vi "Autonomous Independent.vi"() -> ()   [LabVIEW 2016]
doc: "This VI is called when autonomous begins, and will automatically be terminated when autonomous ends. You can carry out timed or sensor driven robot movement independently without needing to return to the caller."
uses:
  <vilib>/Rock Robotics/WPI/Solenoid/WPI_SolenoidValue.ctl
  <vilib>/Rock Robotics/WPI/SafetyOutput/WPI_SafetyOutputConfigMenu.ctl
  <vilib>/Rock Robotics/WPI/Utilities/WPI_GetSetVariantRefNum.vi
  <vilib>/Rock Robotics/Network Tables/NT Read String.vi
  <vilib>/Rock Robotics/Network Tables/NT Write Numeric Array.vi
  <vilib>/Rock Robotics/WPI/Ultrasonic/WPI_SonarMB1010AnalogRefNum Registry Get.vi
  <vilib>/Rock Robotics/WPI/RobotDrive/WPI_RobotDriveArcadeDrive_Standard(NoSaturation).vi
  <vilib>/Rock Robotics/WPI/Solenoid/WPI_SolenoidSetEnum.vi
  <vilib>/addons/control/pid/pid.llb/PID (DBL).vi
  <vilib>/Rock Robotics/WPI/Ultrasonic/WPI_SonarMB1010AnalogGetRange.vi
  <vilib>/Rock Robotics/WPI/ThirdParty/Sensors/ADIS16448 IMU/ADIS16448_IMU.lvlib
  <vilib>/addons/control/pid/NI_PID_pid.lvlib
panel:
  out "Current Movement, for debugging":T1 {"Y Joystick Value" scale=1.0..-1.0; "X Joystick Value" scale=-1.0..1.0}
  in  "Array of robot movements":T2(array[cluster])=[{"X Joystick Value"=0.39393939393939403, "Y Joystick Value"=0.0, "Delay (sec)"=1.0, "Movement Name"="turn"}, {"X Joystick Value"=-0.3737373737373737, "Y Joystick Value"=0.0, "Delay (sec)"=1.0, "Movement Name"="turn back"}] {"Y Joystick Value" scale=1.0..-1.0; "X Joystick Value" scale=-1.0..1.0}
  # "Be sure to right-click and choose Data Operations>>Make Current Value default if you want to save the array values with the VI"
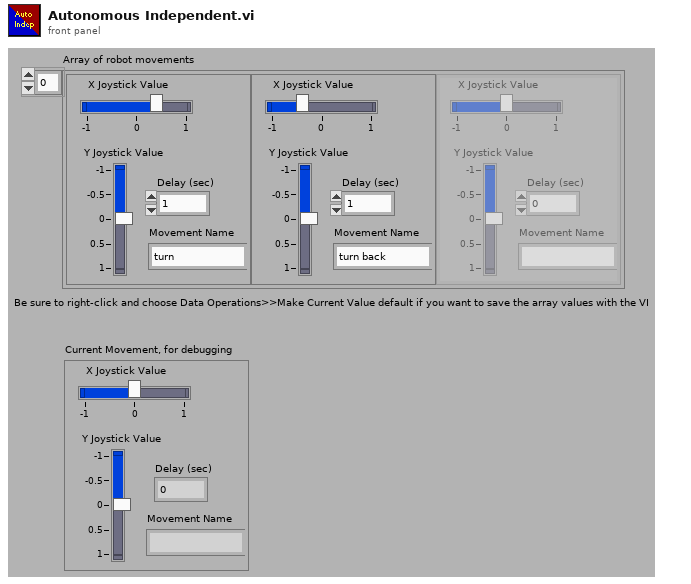
[diagram p1: front panel]
types:
  T1 = cluster{"X Joystick Value":dbl, "Y Joystick Value":dbl, "Delay (sec)":dbl, "Movement Name":string}
  T2 = cluster{"X Joystick Value":dbl, "Y Joystick Value":dbl, "Delay (sec)":dbl, "Movement Name":string}[]
  T3 = typedef "WPI_JoystickDevRef.ctl" = cluster{"Device":T4}
  T4 = typedef "WPI_JoystickDeviceEnum.ctl" = enum16{"USB 0", "USB 1", "USB 2", "USB 3", "USB 4", "USB 5"}
  T5 = typedef "WPI_RobotDriveDevRef.ctl" = cluster{"DevStatus":errorcluster, "Motors[]":T6[], "Square Inputs":bool, "Max Output":dbl}
  T6 = typedef "WPI_MotorControlDeviceRef.ctl" = cluster{"DeviceStatus":errorcluster, "Type":T7, "PWM":cluster{"PWM Channel":T8, "DeadBand":T9}, "CAN":cluster{"Device Number":u8, "SetOutput VI Ref":variant, "GetOutput VI Ref":variant, "Enable VI Ref":variant, "Disable VI Ref":variant, "Data":variant}, "Invert":bool}
  T7 = typedef "WPI_MotorControlType.ctl" = enum16{"PWM", "CAN"}
  T8 = typedef "FPGA_DIOPWMChannel.ctl" = enum8{"PWM 0", "PWM 1", "PWM 2", "PWM 3", "PWM 4", "PWM 5", "PWM 6", "PWM 7", "PWM 8", "PWM 9", "PWM MXP 0", "PWM MXP 1", "PWM MXP 2", "PWM MXP 3", "PWM MXP 4", "PWM MXP 5", "PWM MXP 6", "PWM MXP 7", "PWM MXP 8", "PWM MXP 9", "Invalid"}
  T9 = typedef "WPI_PWMDeadband.ctl" = cluster{"Name":string, "maxPositivePwm":i32, "minPositivePwm":i32, "centerPwm":i32, "maxNegativePwm":i32, "minNegativePwm":i32, "angularRange":u16}
  T10 = typedef "WPI_SonarMB1010AnalogDeviceRef.ctl" = cluster{"AIDeviceRef":T11, "Scaling factor (V/in)":dbl, "Average Bits":u8}
  T11 = typedef "WPI_AnalogChannelDevRef.ctl" = cluster{"DevStatus":errorcluster, "Analog Channel":T12}
  T12 = typedef "FPGA_AIChannel.ctl" = enum8{"AI 0", "AI 1", "AI 2", "AI 3", "AI MXP 0", "AI MXP 1", "AI MXP 2", "AI MXP 3", "Invalid"}
  T13 = typedef "WPI_SolenoidDevRef.ctl" = cluster{"DevStatus":errorcluster, "Pneumatics Control Module":u8, "Forward Solenoid Channel":T14, "Reverse Solenoid Channel":T14}
  T14 = typedef "WPI_SolenoidChannel.ctl" = enum8{"Solenoid 0", "Solenoid 1", "Solenoid 2", "Solenoid 3", "Solenoid 4", "Solenoid 5", "Solenoid 6", "Solenoid 7", "Invalid"}
  T15 = typedef "ADIS16448_IMU.lvlib/ADI_IMU_ADIS16448_InterruptDevRef.ctl" = cluster{"ADI IMU DevRef":T16, "InterruptRef":T18}
  T16 = typedef "ADIS16448_IMU.lvlib/ADI_IMU_ADIS16448_IMUDevRef.ctl" = cluster{"DevStatus":errorcluster, "Handle":i32, "SPI Bus":T17, "Device Found":bool, "Device Ready":bool, "Yaw Axis":enum16{"X", "Y", "Z"}, "AHRS Algorithm":enum16{"Complementary", "Madgwick"}, "Serial":u16, "Lot ID 2":u16, "Lot ID 1":u16, "Product ID":u16}
  T17 = typedef "spi_bus.ctl" = enum16{"SPI On-Board, CS0", "SPI On-Board, CS1", "SPI On-Board, CS2", "SPI On-Board, CS3", "SPI MXP", "Invalid"}
  T18 = typedef "WPI_InterruptRef.ctl" = cluster{"DevStatus":errorcluster, "InterruptIndex":T19}
  T19 = typedef "FPGA_InterruptIndex.ctl" = enum8{"0", "1", "2", "3", "4", "5", "6", "7", "Invalid"}
  T20 = typedef "WPI_SolenoidValue.ctl" = enum16{"Off", "On", "Forward", "Reverse"}
  T21 = typedef "WPI_SafetyOutputConfigMenu.ctl" = enum16{"Enable", "Disable"}
  T22 = cluster{"proportional gain (Kc)":dbl, "integral time (Ti, min)":dbl, "derivative time (Td, min)":dbl}
  T23 = cluster{"X Angle":dbl, "Y Angle":dbl, "Z Angle":dbl}
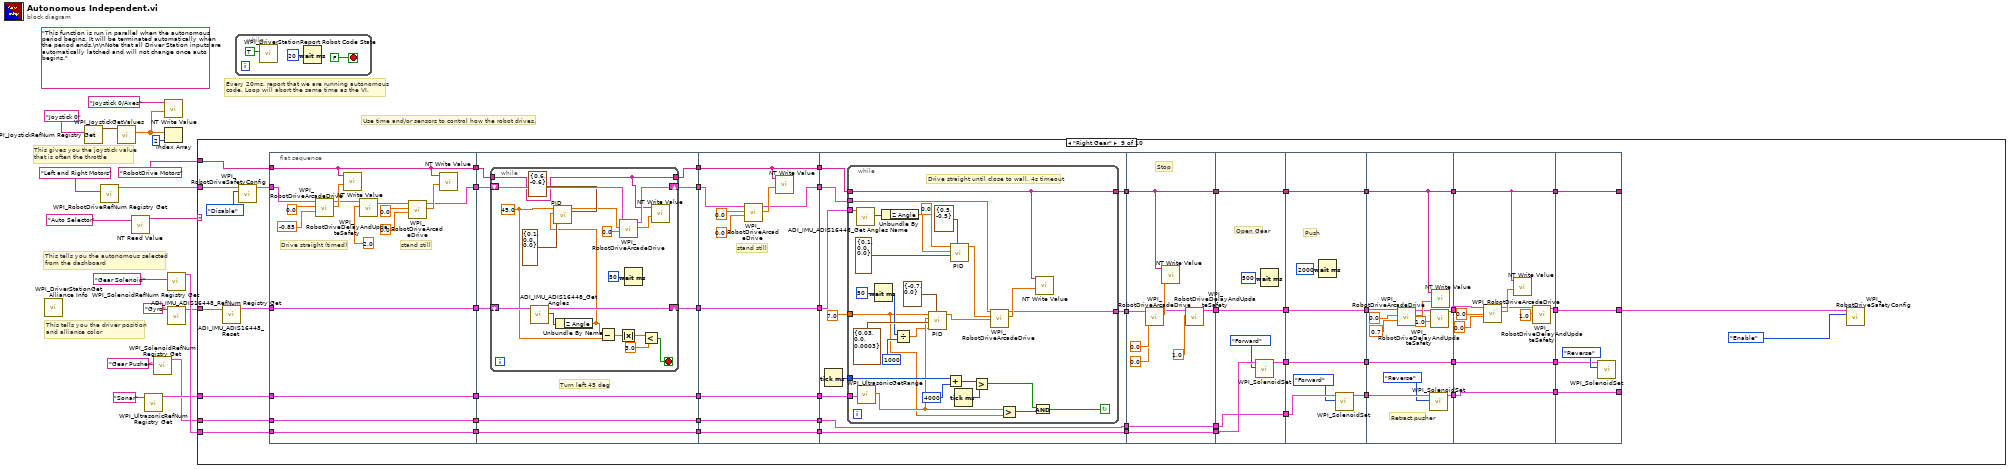
[diagram p0: block diagram]
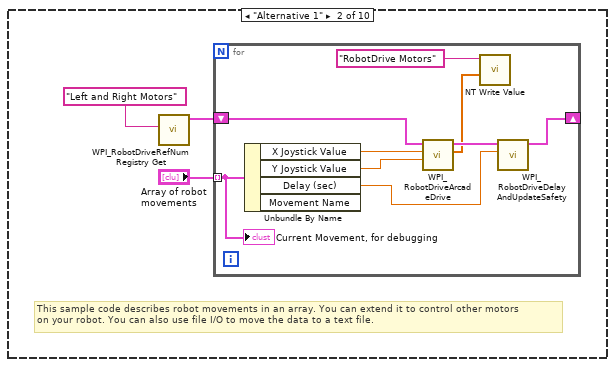
[diagram p3: hidden frame]
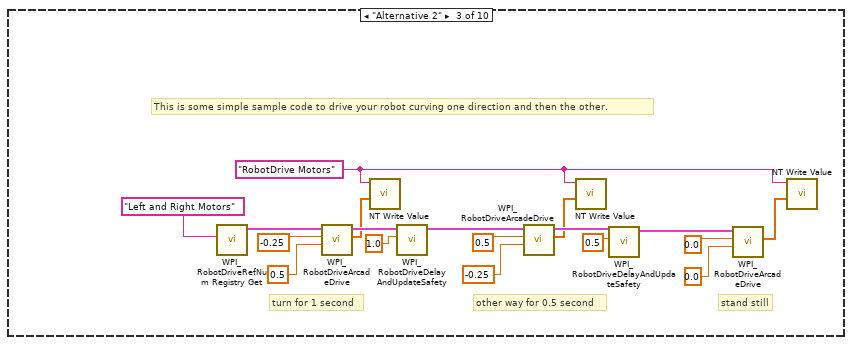
[diagram p4: hidden frame]
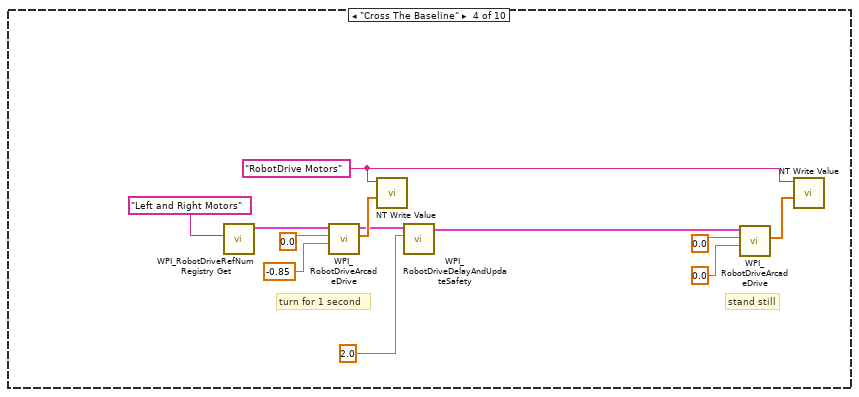
[diagram p5: hidden frame]
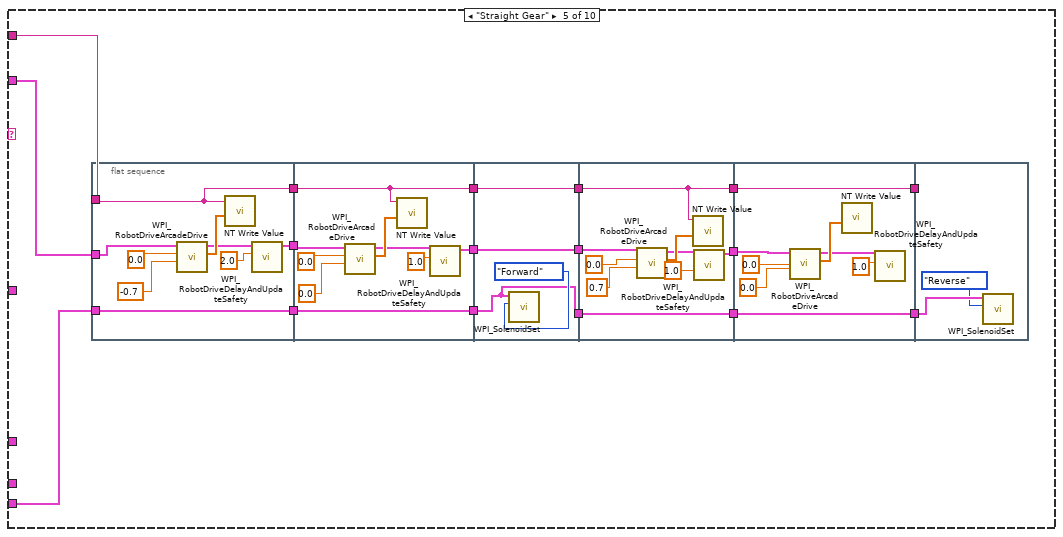
[diagram p6: hidden frame]
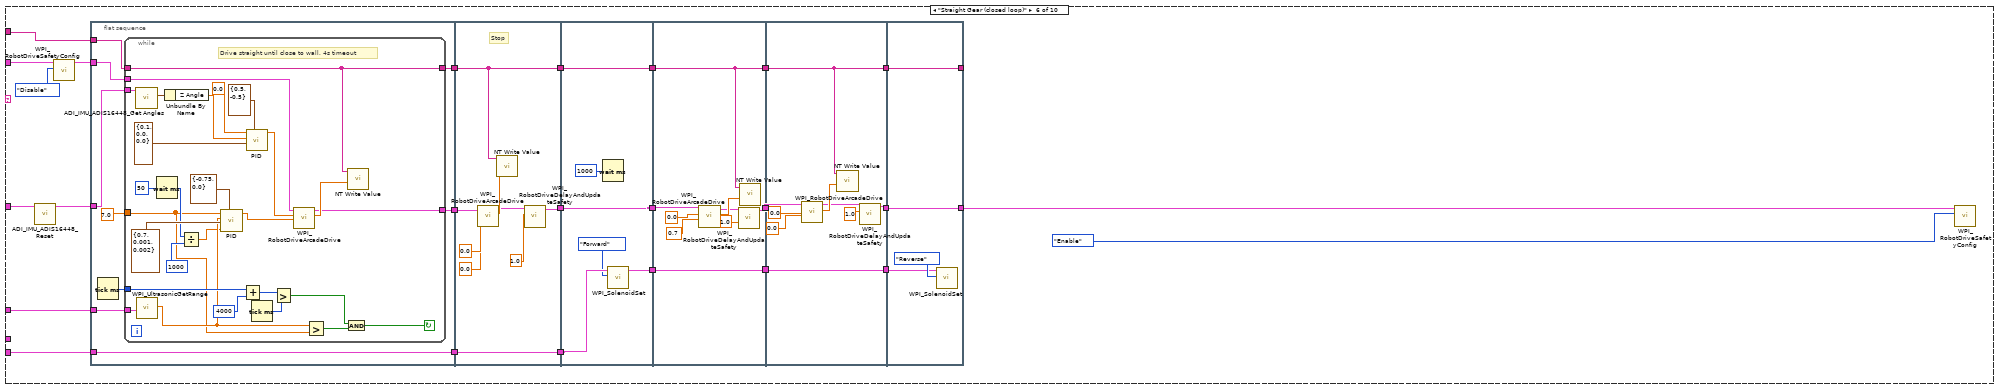
[diagram p7: hidden frame]
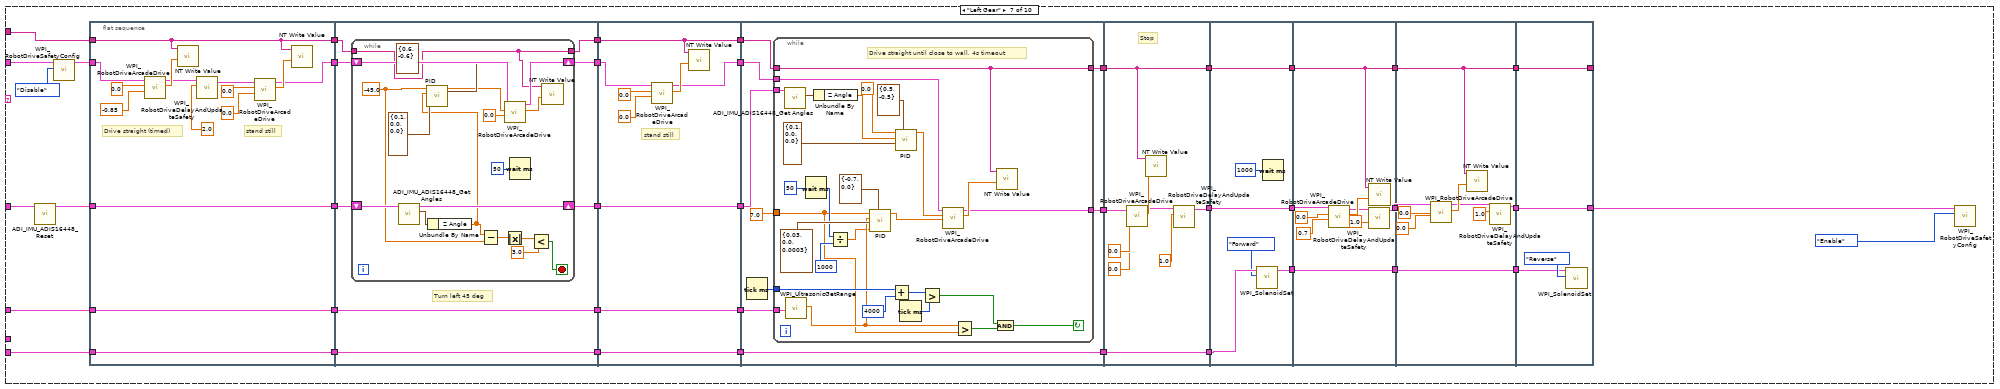
[diagram p8: hidden frame]
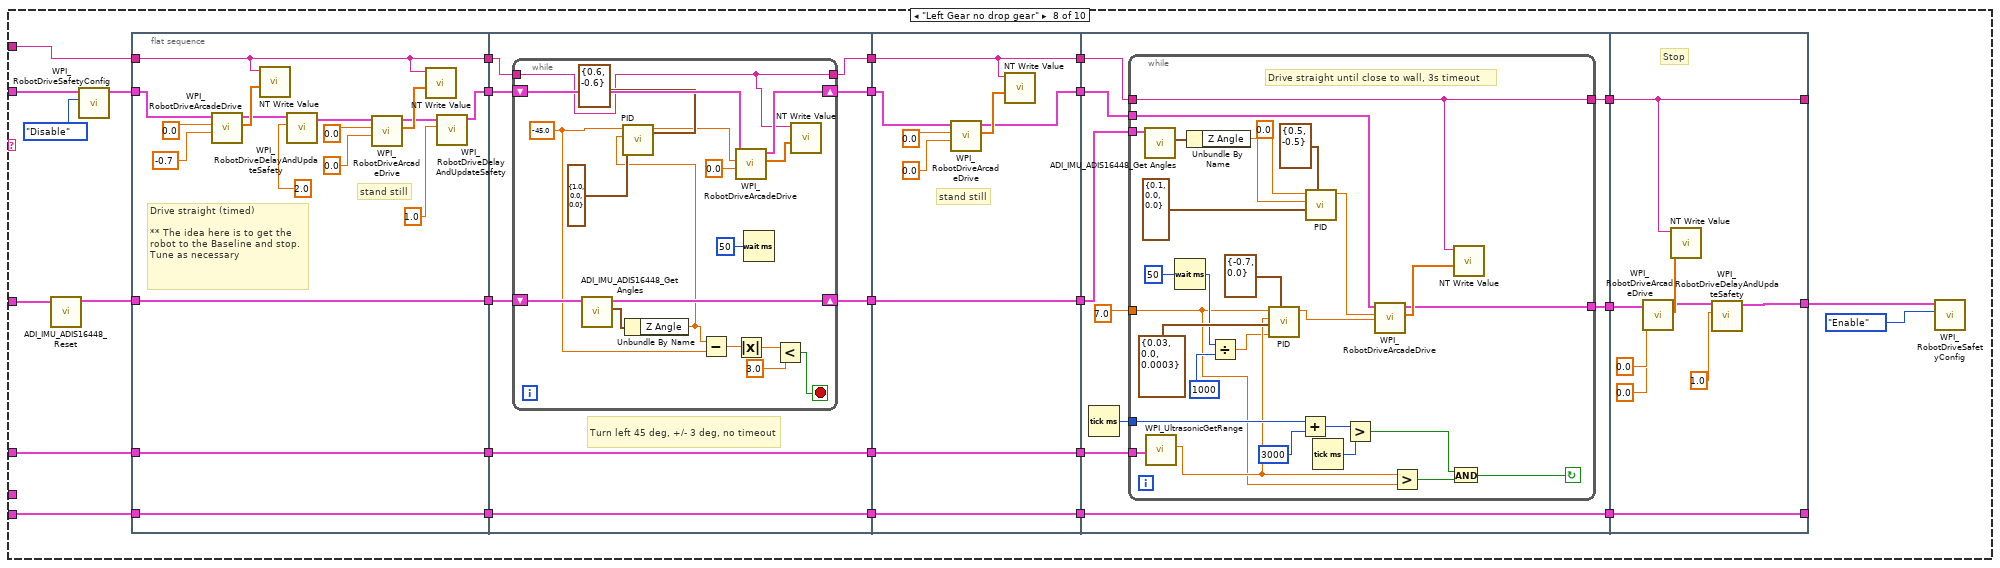
[diagram p9: hidden frame]
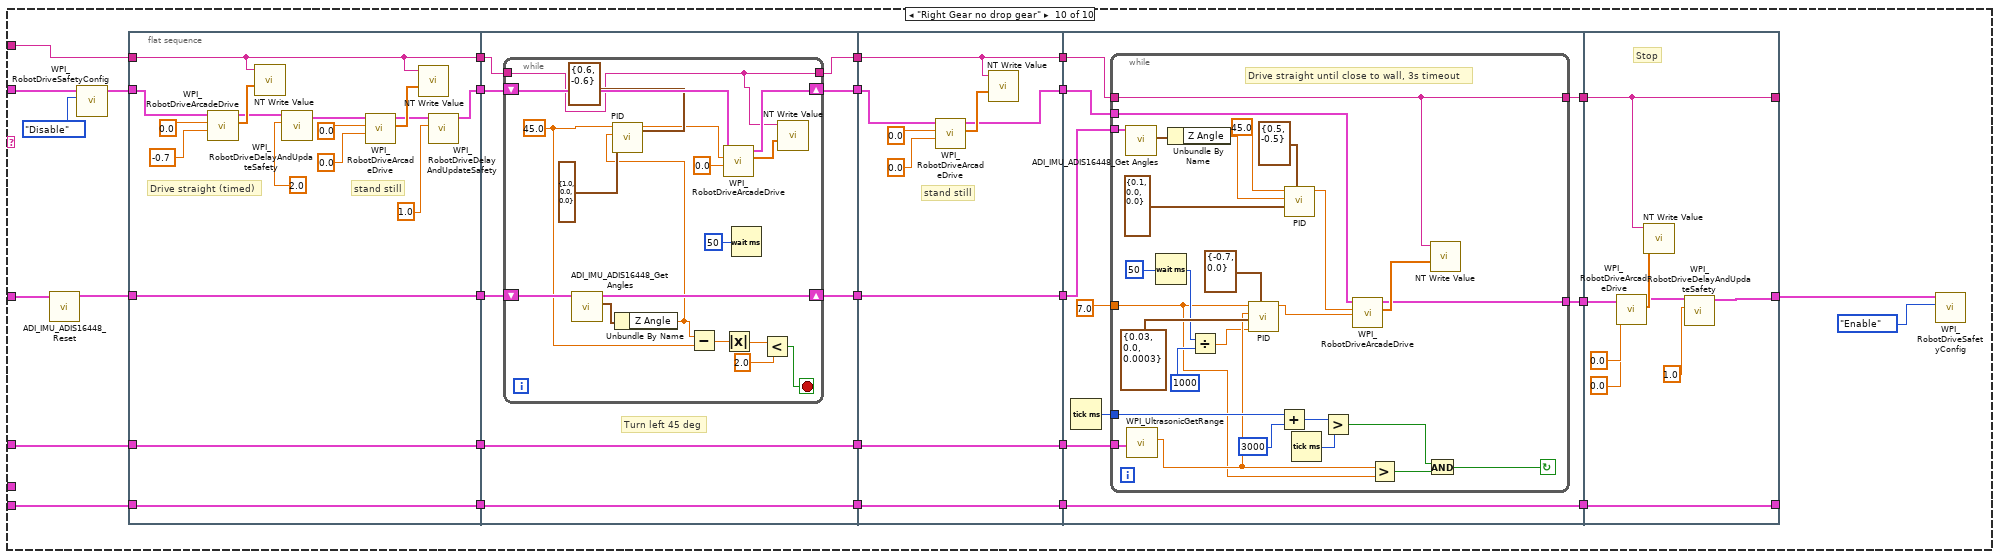
[diagram p10: hidden frame]
diagram:
  (unwired) "This function is run in parallel when the autonomous period begins. It will be terminated automatically when the period ends.\n\nNote that all Driver Station inputs are automatically latched and will not change once auto begins."
  # "This tells you the autonomous selected\nfrom the dashboard"
  # "Every 20ms, report that we are running autonomous\ncode. Loop will abort the same time as the VI."
  # "This gives you the joystick value\nthat is often the throttle"
  # "Use time and/or sensors to control how the robot drives."
  # "This tells you the driver position\nand alliance color"
  n1 = call <vilib>:"WPI_DriverStationGet Alliance Info.vi"() -> ()  [unwired: 12 out]
  n2 = call <vilib>:"WPI_JoystickRefNum Registry Get.vi"("refnum name"="Joystick 0") -> ("JoystickDevRef"=w17:T3)  [unwired: 1 in, 9 out]
  n3 = call <vilib>:"WPI_RobotDriveRefNum Registry Get.vi"("refnum name"="Left and Right Motors") -> ("RobotDriveDevRef"=w10:T5)  [unwired: 1 in, 9 out]
  n4 = call <vilib>:"WPI_JoystickGetValues.vi"("JoystickDevRef"=w17) -> ("Axes"=w13:dbl[])  [unwired: 6 in, 4 out]
  n5 = call-poly <vilib>:"NT Read Value.vi"("Name"="Auto Selector") -> ("String"=w14:string)  [unwired: 9 in, 1 out]
  n6 = call-poly <vilib>:"WPI_UltrasonicRefNum Registry Get.vi"("refnum name"="Sonar") -> ("SonarMB1010AnalogDevRef"=w3:T10)  [unwired: 9 in, 1 out]
  n7 = call <vilib>:"WPI_SolenoidRefNum Registry Get.vi"("refnum name"="Gear Pusher") -> ("SolenoidDevRef"=w1:T13)  [unwired: 9 in, 1 out]
  n8 = call-poly <vilib>:"NT Write Value.vi"("Numeric Array"=w13, "Name"="Joystick 0/Axes") -> ()  [unwired: 9 in, 1 out]
  n9 = Index Array(array=w13, index=2) -> ()  [unwired: 1 out]
  n10 = call <vilib>:"WPI_SolenoidRefNum Registry Get.vi"("refnum name"="Gear Solenoid") -> ("SolenoidDevRef"=w7:T13)  [unwired: 9 in, 1 out]
  n11 = call <vilib>:"ADI_IMU_ADIS16448_RefNum Registry Get.vi"("refnum name"="Gyro") -> ("ADI IMU Interrupt DevRef"=w5:T15)  [unwired: 9 in, 1 out]
  n12 = case shown="\"Right Gear\"" w14 {
    tunnel: w10 -> [_ _ _ _ w77 w138 w251 w402 w552 w721]
    tunnel: "RobotDrive Motors" ("Name") -> [_ _ _ _ w76 w140 w253 w404 w554 w723]
    tunnel: w7 -> [_ _ _ _ w71 w139 w252 w403 w553 w722]
    tunnel: w5 -> [_ _ _ _ _ w143 w256 w407 w557 w726]
    tunnel: w3 -> [_ _ _ _ _ w142 w255 w406 w556 w725]
    tunnel: w1 -> [_ _ _ _ _ _ _ _ w520 _]
    frame Default {
      # "You can put your main auto here, or you can right-click on the case and make any\nother frame be the default case."
      # "This is the frame that will execute if no selection is made, or if it is not recognized"
    }
    frame "Alternative 1" {
      # "This sample code describes robot movements in an array. You can extend it to control other motors\non your robot. You can also use file I/O to move the data to a text file."
      n13 = call <vilib>:"WPI_RobotDriveRefNum Registry Get.vi"("refnum name"="Left and Right Motors") -> ("RobotDriveDevRef"=w20:T5)  [unwired: 1 in, 9 out]
      n14 = for {
        shift-right: [w28] -> _
        shift-left: w20 -> [w29]
        tunnel: "Array of robot movements" -> [w24] mode=indexing
        n15 = Unbundle By Name(w24) -> ("X Joystick Value"=w27:dbl, "Y Joystick Value"=w26:dbl, "Delay (sec)"=w25:dbl)  [unwired: 1 out]
        n16 = call-poly <vilib>:"WPI_RobotDriveArcadeDrive.vi"("Y axis value"=w26, "X axis value"=w27, "RobotDriveDevRef"=w29) -> ("Motor Values"=w22:dbl[], "RobotDriveDevRef"=w30:T5)  [unwired: 1 in, 6 out]
        n17 = call-poly <vilib>:"NT Write Value.vi"("Numeric Array"=w22, "Name"="RobotDrive Motors") -> ()  [unwired: 9 in, 1 out]
        n18 = call <vilib>:"WPI_RobotDriveDelayAndUpdateSafety.vi"("Delay (s)"=w25, "RobotDriveDevRef"=w30) -> ("RobotDriveDevRef 2"=w28:T5)  [unwired: 8 in, 1 out]
        "Current Movement, for debugging" <- w24
      }
    }
    frame "Alternative 2" {
      w32 = "RobotDrive Motors" ("Name")
      # "This is some simple sample code to drive your robot curving one direction and then the other."
      # "stand still"
      # "other way for 0.5 second"
      # "turn for 1 second"
      n19 = call <vilib>:"WPI_RobotDriveRefNum Registry Get.vi"("refnum name"="Left and Right Motors") -> ("RobotDriveDevRef"=w48:T5)  [unwired: 1 in, 9 out]
      n20 = call-poly <vilib>:"WPI_RobotDriveArcadeDrive.vi"("Y axis value"=0.5 ("X axis value"), "X axis value"=-0.25, "RobotDriveDevRef"=w48) -> ("Motor Values"=w31:dbl[], "RobotDriveDevRef"=w41:T5)  [unwired: 1 in, 6 out]
      n21 = call-poly <vilib>:"NT Write Value.vi"("Numeric Array"=w31, "Name"=w32) -> ()  [unwired: 9 in, 1 out]
      n22 = call <vilib>:"WPI_RobotDriveDelayAndUpdateSafety.vi"("Delay (s)"=1.0, "RobotDriveDevRef"=w41) -> ("RobotDriveDevRef 2"=w42:T5)  [unwired: 8 in, 1 out]
      n23 = call-poly <vilib>:"WPI_RobotDriveArcadeDrive.vi"("Y axis value"=-0.25 ("X axis value"), "X axis value"=0.5, "RobotDriveDevRef"=w42) -> ("Motor Values"=w33:dbl[], "RobotDriveDevRef"=w43:T5)  [unwired: 1 in, 6 out]
      n24 = call-poly <vilib>:"NT Write Value.vi"("Numeric Array"=w33, "Name"=w32) -> ()  [unwired: 9 in, 1 out]
      n25 = call <vilib>:"WPI_RobotDriveDelayAndUpdateSafety.vi"("Delay (s)"=0.5, "RobotDriveDevRef"=w43) -> ("RobotDriveDevRef 2"=w44:T5)  [unwired: 8 in, 1 out]
      n26 = call-poly <vilib>:"WPI_RobotDriveArcadeDrive.vi"("Y axis value"=0.0 ("X axis value"), "X axis value"=0.0, "RobotDriveDevRef"=w44) -> ("Motor Values"=w34:dbl[])  [unwired: 1 in, 7 out]
      n27 = call-poly <vilib>:"NT Write Value.vi"("Numeric Array"=w34, "Name"=w32) -> ()  [unwired: 9 in, 1 out]
    }
    frame "Cross The Baseline" {
      w59 = "RobotDrive Motors" ("Name")
      # "stand still"
      # "turn for 1 second"
      n28 = call <vilib>:"WPI_RobotDriveRefNum Registry Get.vi"("refnum name"="Left and Right Motors") -> ("RobotDriveDevRef"=w50:T5)  [unwired: 1 in, 9 out]
      n29 = call-poly <vilib>:"WPI_RobotDriveArcadeDrive.vi"("Y axis value"=-0.85 ("X axis value"), "X axis value"=0.0, "RobotDriveDevRef"=w50) -> ("Motor Values"=w60:dbl[], "RobotDriveDevRef"=w53:T5)  [unwired: 1 in, 6 out]
      n30 = call-poly <vilib>:"NT Write Value.vi"("Numeric Array"=w60, "Name"=w59) -> ()  [unwired: 9 in, 1 out]
      n31 = call <vilib>:"WPI_RobotDriveDelayAndUpdateSafety.vi"("Delay (s)"=2.0, "RobotDriveDevRef"=w53) -> ("RobotDriveDevRef 2"=w49:T5)  [unwired: 8 in, 1 out]
      n32 = call-poly <vilib>:"WPI_RobotDriveArcadeDrive.vi"("Y axis value"=0.0 ("X axis value"), "X axis value"=0.0, "RobotDriveDevRef"=w49) -> ("Motor Values"=w58:dbl[])  [unwired: 1 in, 7 out]
      n33 = call-poly <vilib>:"NT Write Value.vi"("Numeric Array"=w58, "Name"=w59) -> ()  [unwired: 9 in, 1 out]
    }
    frame "Straight Gear" {
      n34 = flat-sequence {
        tunnel: w77 -> [w81]
        tunnel: w76 -> [w79]
        tunnel: [w80] -> w75
        tunnel: [w79] -> w74
        tunnel: w71 -> [w78]
        tunnel: [w78] -> w70
        tunnel: w75 -> [w90]
        tunnel: w74 -> [w89]
        tunnel: [w89] -> w73
        tunnel: w70 -> [w88]
        tunnel: [w88] -> w69
        tunnel: [w87] -> w66
        tunnel: w73 -> [w99]
        tunnel: [w99] -> w72
        tunnel: w69 -> [w96]
        tunnel: w66 -> [w97]
        tunnel: [w97] -> w65
        tunnel: [w96] -> w63
        tunnel: w72 -> [w105]
        tunnel: [w105] -> w68
        tunnel: w65 -> [w104]
        tunnel: [w101] -> w64
        tunnel: w63 -> [w103]
        tunnel: [w103] -> w62
        tunnel: w68 -> [w116]
        tunnel: [w116] -> w67
        tunnel: w64 -> [w110]
        tunnel: w62 -> [w109]
        tunnel: [w109] -> w61
        tunnel: w67 -> [_]
        tunnel: w61 -> [w118]
        frame #0 {
          n35 = call-poly <vilib>:"WPI_RobotDriveArcadeDrive.vi"("Y axis value"=-0.7 ("X axis value"), "X axis value"=0.0, "RobotDriveDevRef"=w81) -> ("Motor Values"=w86:dbl[], "RobotDriveDevRef"=w83:T5)  [unwired: 1 in, 6 out]
          n36 = call-poly <vilib>:"NT Write Value.vi"("Numeric Array"=w86, "Name"=w79) -> ()  [unwired: 9 in, 1 out]
          n37 = call <vilib>:"WPI_RobotDriveDelayAndUpdateSafety.vi"("Delay (s)"=2.0, "RobotDriveDevRef"=w83) -> ("RobotDriveDevRef 2"=w80:T5)  [unwired: 8 in, 1 out]
        }
        frame #1 {
          n38 = call-poly <vilib>:"WPI_RobotDriveArcadeDrive.vi"("Y axis value"=0.0 ("X axis value"), "X axis value"=0.0, "RobotDriveDevRef"=w90) -> ("Motor Values"=w95:dbl[], "RobotDriveDevRef"=w92:T5)  [unwired: 1 in, 6 out]
          n39 = call-poly <vilib>:"NT Write Value.vi"("Numeric Array"=w95, "Name"=w89) -> ()  [unwired: 9 in, 1 out]
          n40 = call <vilib>:"WPI_RobotDriveDelayAndUpdateSafety.vi"("Delay (s)"=1.0, "RobotDriveDevRef"=w92) -> ("RobotDriveDevRef 2"=w87:T5)  [unwired: 8 in, 1 out]
        }
        frame #2 {
          n41 = call-poly <vilib>:"WPI_SolenoidSet.vi"("Value"=WPI_SolenoidValue."Forward", "SolenoidDevRef"=w96) -> ()  [unwired: 8 in, 2 out]
        }
        frame #3 {
          w100 = 1.0 ("Delay (s)")
          n42 = call-poly <vilib>:"WPI_RobotDriveArcadeDrive.vi"("Y axis value"=0.7 ("X axis value"), "X axis value"=0.0, "RobotDriveDevRef"=w104) -> ("Motor Values"=w108:dbl[], "RobotDriveDevRef"=w102:T5)  [unwired: 1 in, 6 out]
          n43 = call-poly <vilib>:"NT Write Value.vi"("Numeric Array"=w108, "Name"=w105) -> ()  [unwired: 9 in, 1 out]
          n44 = call <vilib>:"WPI_RobotDriveDelayAndUpdateSafety.vi"("Feed time (s)"=w100, "Delay (s)"=w100, "RobotDriveDevRef"=w102) -> ("RobotDriveDevRef 2"=w101:T5)  [unwired: 7 in, 1 out]
        }
        frame #4 {
          n45 = call-poly <vilib>:"WPI_RobotDriveArcadeDrive.vi"("Y axis value"=0.0 ("X axis value"), "X axis value"=0.0, "RobotDriveDevRef"=w110) -> ("Motor Values"=w115:dbl[], "RobotDriveDevRef"=w113:T5)  [unwired: 1 in, 6 out]
          n46 = call-poly <vilib>:"NT Write Value.vi"("Numeric Array"=w115) -> ()  [unwired: 10 in, 1 out]
          n47 = call <vilib>:"WPI_RobotDriveDelayAndUpdateSafety.vi"("Delay (s)"=1.0, "RobotDriveDevRef"=w113) -> ()  [unwired: 8 in, 2 out]
        }
        frame #5 {
          n48 = call-poly <vilib>:"WPI_SolenoidSet.vi"("Value"=WPI_SolenoidValue."Reverse", "SolenoidDevRef"=w118) -> ()  [unwired: 8 in, 2 out]
        }
      }
    }
    frame "Straight Gear (closed loop)" {
      n49 = call <vilib>:"ADI_IMU_ADIS16448_Reset.vi"("ADI IMU Interrupt DevRef"=w143) -> ("ADI IMU Interrupt DevRef Out"=w141:T15)  [unwired: 9 in, 1 out]
      n50 = call <vilib>:"WPI_RobotDriveSafetyConfig.vi"("mode"=WPI_SafetyOutputConfigMenu."Disable", "RobotDriveDevRef"=w138) -> ("RobotDriveDevRef"=w137:T5)  [unwired: 8 in, 1 out]
      n51 = flat-sequence {
        tunnel: w142 -> [w152]
        tunnel: w141 -> [w145]
        tunnel: w140 -> [w150]
        tunnel: w137 -> [w149]
        tunnel: w139 -> [w144]
        tunnel: [w148] -> w133
        tunnel: [w147] -> w132
        tunnel: [w144] -> w129
        tunnel: w133 -> [w188]
        tunnel: w132 -> [w184]
        tunnel: [w181] -> w131
        tunnel: [w184] -> w130
        tunnel: w129 -> [w183]
        tunnel: [w183] -> w128
        tunnel: w131 -> [w190]
        tunnel: w130 -> [w194]
        tunnel: w128 -> [w193]
        tunnel: [w190] -> w127
        tunnel: [w194] -> w126
        tunnel: [w192] -> w125
        tunnel: w127 -> [w195]
        tunnel: w126 -> [w196]
        tunnel: w125 -> [w203]
        tunnel: [w197] -> w124
        tunnel: [w196] -> w123
        tunnel: [w203] -> w122
        tunnel: w124 -> [w206]
        tunnel: w123 -> [w204]
        tunnel: w122 -> [w212]
        tunnel: [w205] -> w121
        tunnel: [w204] -> w120
        tunnel: [w212] -> w119
        tunnel: [w215] -> _
        tunnel: [w216] -> w135
        tunnel: w121 -> [w216]
        tunnel: w120 -> [w215]
        tunnel: w119 -> [w213]
        frame #0 {
          n52 = Tick Count (ms)() -> (millisecond timer value=w151:u32)
          n53 = while {
            tunnel: w152 -> [w179]
            tunnel: w151 -> [w177]
            tunnel: w150 -> [w166]
            tunnel: w149 -> [w171]
            tunnel: [w170] -> w148
            tunnel: [w166] -> w147
            tunnel: 7.0 ("setpoint") -> [w161]
            tunnel: w145 -> [w160]
            stop <- w163 continue-if-true
            w169 = u32 50 ("milliseconds to wait")
            # "Drive straight until close to wall, 4s timeout"
            n54 = call <vilib>:"ADI_IMU_ADIS16448_Get Angles.vi"("ADI IMU Interrupt DevRef"=w160) -> ("IMU Angles Out"=w155:T23)  [unwired: 7 in, 3 out]
            n55 = call-poly <vilib>:"WPI_UltrasonicGetRange.vi"("SonarMB1010AnalogDevRef"=w179) -> ("Distance"=w173:dbl)  [unwired: 8 in, 2 out]
            n56 = Wait (ms)(milliseconds to wait=w169) -> ()  [unwired: 1 out]
            n57 = Unbundle By Name(w155) -> ("Z Angle"=w154:dbl)
            n58 = Divide(x=w169, y=u32 1000) -> (x/y=w167:dbl)
            n59 = call-poly <vilib>:"PID.vi"("output range"=cluster{"output high":dbl, "output low":dbl} {"output high"=-0.75, "output low"=0.0}, "dt (s)"=w167, "PID gains"=T22 {"proportional gain (Kc)"=0.7, "integral time (Ti, min)"=0.001, "derivative time (Td, min)"=0.002}, "process variable"=w173, "setpoint"=w161) -> ("output"=w153:dbl)  [unwired: 5 in, 1 out]
            n60 = Add(x=w177, y=u32 4000) -> (x+y=w165:u32)
            n61 = call-poly <vilib>:"PID.vi"("output range"=cluster{"output high":dbl, "output low":dbl} {"output high"=0.5, "output low"=-0.5}, "PID gains"=T22 {"proportional gain (Kc)"=0.1, "integral time (Ti, min)"=0.0, "derivative time (Td, min)"=0.0}, "process variable"=w154, "setpoint"=0.0) -> ("output"=w157:dbl)  [unwired: 6 in, 1 out]
            n62 = Tick Count (ms)() -> (millisecond timer value=w164:u32)
            n63 = Greater?(x=w165, y=w164) -> (0:w162:bool)
            n64 = call-poly <vilib>:"WPI_RobotDriveArcadeDrive.vi"("Y axis value"=w153, "X axis value"=w157, "RobotDriveDevRef"=w171) -> ("Motor Values"=w172:dbl[], "RobotDriveDevRef"=w170:T5)  [unwired: 6 in, 1 out]
            n65 = Greater?(x=w173, y=w161) -> (0:w178:bool)
            n66 = And(x=w162, y=w178) -> (x .and. y?=w163:bool)
            n67 = call-poly <vilib>:"NT Write Value.vi"("Numeric Array"=w172, "Name"=w166) -> ()  [unwired: 9 in, 1 out]
          }
        }
        frame #1 {
          # "Stop"
          n68 = call-poly <vilib>:"WPI_RobotDriveArcadeDrive.vi"("Y axis value"=0.0, "X axis value"=0.0, "RobotDriveDevRef"=w188) -> ("Motor Values"=w187:dbl[], "RobotDriveDevRef"=w182:T5)  [unwired: 6 in, 1 out]
          n69 = call-poly <vilib>:"NT Write Value.vi"("Numeric Array"=w187, "Name"=w184) -> ()  [unwired: 9 in, 1 out]
          n70 = call <vilib>:"WPI_RobotDriveDelayAndUpdateSafety.vi"("Delay (s)"=1.0, "RobotDriveDevRef"=w182) -> ("RobotDriveDevRef 2"=w181:T5)  [unwired: 8 in, 1 out]
        }
        frame #2 {
          n71 = Wait (ms)(milliseconds to wait=u32 1000) -> ()  [unwired: 1 out]
          n72 = call-poly <vilib>:"WPI_SolenoidSet.vi"("Value"=WPI_SolenoidValue."Forward", "SolenoidDevRef"=w193) -> ("SolenoidDevRef"=w192:T13)  [unwired: 8 in, 1 out]
        }
        frame #3 {
          n73 = call-poly <vilib>:"WPI_RobotDriveArcadeDrive.vi"("Y axis value"=0.7 ("X axis value"), "X axis value"=0.0, "RobotDriveDevRef"=w195) -> ("Motor Values"=w202:dbl[], "RobotDriveDevRef"=w199:T5)  [unwired: 1 in, 6 out]
          n74 = call <vilib>:"WPI_RobotDriveDelayAndUpdateSafety.vi"("Delay (s)"=1.0, "RobotDriveDevRef"=w199) -> ("RobotDriveDevRef 2"=w197:T5)  [unwired: 8 in, 1 out]
          n75 = call-poly <vilib>:"NT Write Value.vi"("Numeric Array"=w202, "Name"=w196) -> ()  [unwired: 9 in, 1 out]
        }
        frame #4 {
          n76 = call-poly <vilib>:"WPI_RobotDriveArcadeDrive.vi"("Y axis value"=0.0 ("X axis value"), "X axis value"=0.0, "RobotDriveDevRef"=w206) -> ("Motor Values"=w211:dbl[], "RobotDriveDevRef"=w209:T5)  [unwired: 1 in, 6 out]
          n77 = call-poly <vilib>:"NT Write Value.vi"("Numeric Array"=w211, "Name"=w204) -> ()  [unwired: 9 in, 1 out]
          n78 = call <vilib>:"WPI_RobotDriveDelayAndUpdateSafety.vi"("Delay (s)"=1.0, "RobotDriveDevRef"=w209) -> ("RobotDriveDevRef 2"=w205:T5)  [unwired: 8 in, 1 out]
        }
        frame #5 {
          n79 = call-poly <vilib>:"WPI_SolenoidSet.vi"("Value"=WPI_SolenoidValue."Reverse", "SolenoidDevRef"=w213) -> ()  [unwired: 8 in, 2 out]
        }
      }
      n80 = call <vilib>:"WPI_RobotDriveSafetyConfig.vi"("mode"=WPI_SafetyOutputConfigMenu."Enable", "RobotDriveDevRef"=w135) -> ()  [unwired: 8 in, 2 out]
    }
    frame "Left Gear" {
      n81 = call <vilib>:"ADI_IMU_ADIS16448_Reset.vi"("ADI IMU Interrupt DevRef"=w256) -> ("ADI IMU Interrupt DevRef Out"=w254:T15)  [unwired: 9 in, 1 out]
      n82 = call <vilib>:"WPI_RobotDriveSafetyConfig.vi"("mode"=WPI_SafetyOutputConfigMenu."Disable", "RobotDriveDevRef"=w251) -> ("RobotDriveDevRef"=w250:T5)  [unwired: 8 in, 1 out]
      n83 = flat-sequence {
        tunnel: w252 -> [w269]
        tunnel: w250 -> [w259]
        tunnel: w253 -> [w258]
        tunnel: w254 -> [w270]
        tunnel: w255 -> [w271]
        tunnel: [w271] -> w221
        tunnel: [w270] -> w220
        tunnel: [w258] -> w219
        tunnel: [w257] -> w218
        tunnel: [w269] -> w217
        tunnel: [w279] -> w226
        tunnel: [w274] -> w225
        tunnel: [w272] -> w224
        tunnel: [w276] -> w223
        tunnel: [w278] -> w222
        tunnel: w221 -> [w279]
        tunnel: w220 -> [w275]
        tunnel: w219 -> [w273]
        tunnel: w218 -> [w277]
        tunnel: w217 -> [w278]
        tunnel: [w306] -> w231
        tunnel: [w305] -> w230
        tunnel: [w300] -> w229
        tunnel: [w298] -> w228
        tunnel: [w304] -> w227
        tunnel: w226 -> [w306]
        tunnel: w225 -> [w305]
        tunnel: w224 -> [w300]
        tunnel: w223 -> [w299]
        tunnel: w222 -> [w304]
        tunnel: [w311] -> w246
        tunnel: [w310] -> w245
        tunnel: [w307] -> w242
        tunnel: w231 -> [w315]
        tunnel: w230 -> [w308]
        tunnel: w229 -> [w313]
        tunnel: w228 -> [w312]
        tunnel: w227 -> [w307]
        tunnel: w246 -> [w351]
        tunnel: w245 -> [w347]
        tunnel: [w344] -> w244
        tunnel: [w347] -> w243
        tunnel: w242 -> [w346]
        tunnel: [w346] -> w241
        tunnel: w244 -> [w357]
        tunnel: w243 -> [w356]
        tunnel: w241 -> [w355]
        tunnel: [w357] -> w240
        tunnel: [w356] -> w239
        tunnel: [w354] -> w238
        tunnel: w240 -> [w360]
        tunnel: w239 -> [w358]
        tunnel: w238 -> [w366]
        tunnel: [w359] -> w237
        tunnel: [w358] -> w236
        tunnel: [w366] -> w235
        tunnel: w237 -> [w369]
        tunnel: w236 -> [w367]
        tunnel: w235 -> [w375]
        tunnel: [w368] -> w234
        tunnel: [w367] -> w233
        tunnel: [w375] -> w232
        tunnel: [w378] -> _
        tunnel: [w379] -> w248
        tunnel: w234 -> [w379]
        tunnel: w233 -> [w378]
        tunnel: w232 -> [w376]
        frame #0 {
          # "stand still"
          # "Drive straight (timed)"
          n84 = call-poly <vilib>:"WPI_RobotDriveArcadeDrive.vi"("Y axis value"=-0.85 ("X axis value"), "X axis value"=0.0, "RobotDriveDevRef"=w259) -> ("Motor Values"=w268:dbl[], "RobotDriveDevRef"=w262:T5)  [unwired: 1 in, 6 out]
          n85 = call-poly <vilib>:"NT Write Value.vi"("Numeric Array"=w268, "Name"=w258) -> ()  [unwired: 9 in, 1 out]
          n86 = call <vilib>:"WPI_RobotDriveDelayAndUpdateSafety.vi"("Delay (s)"=2.0, "RobotDriveDevRef"=w262) -> ("RobotDriveDevRef 2"=w260:T5)  [unwired: 8 in, 1 out]
          n87 = call-poly <vilib>:"WPI_RobotDriveArcadeDrive.vi"("Y axis value"=0.0 ("X axis value"), "X axis value"=0.0, "RobotDriveDevRef"=w260) -> ("Motor Values"=w267:dbl[], "RobotDriveDevRef"=w257:T5)  [unwired: 1 in, 6 out]
          n88 = call-poly <vilib>:"NT Write Value.vi"("Numeric Array"=w267, "Name"=w258) -> ()  [unwired: 9 in, 1 out]
        }
        frame #1 {
          # "Turn left 45 deg"
          n89 = while {
            shift-right: [w295] -> w276
            shift-left: w277 -> [w296]
            shift-right: [w292] -> w274
            shift-left: w275 -> [w293]
            tunnel: w273 -> [w286]
            tunnel: [w286] -> w272
            stop <- w280 stop-if-true
            w284 = -45.0 ("setpoint")
            n90 = call <vilib>:"ADI_IMU_ADIS16448_Get Angles.vi"("ADI IMU Interrupt DevRef"=w293) -> ("IMU Angles Out"=w294:T23, "ADI IMU Interrupt DevRef Out"=w292:T15)  [unwired: 7 in, 2 out]
            n91 = Unbundle By Name(w294) -> ("Z Angle"=w285:dbl)
            n92 = call-poly <vilib>:"PID.vi"("output range"=cluster{"output high":dbl, "output low":dbl} {"output high"=0.6, "output low"=-0.6}, "PID gains"=T22 {"proportional gain (Kc)"=0.1, "integral time (Ti, min)"=0.0, "derivative time (Td, min)"=0.0}, "process variable"=w285, "setpoint"=w284) -> ("output"=w289:dbl)  [unwired: 6 in, 1 out]
            n93 = Subtract(x=w285, y=w284) -> (x-y=w283:dbl)
            n94 = call-poly <vilib>:"WPI_RobotDriveArcadeDrive.vi"("Y axis value"=0.0, "X axis value"=w289, "RobotDriveDevRef"=w296) -> ("Motor Values"=w287:dbl[], "RobotDriveDevRef"=w295:T5)  [unwired: 6 in, 1 out]
            n95 = Absolute Value(x=w283) -> (abs(x)=w282:dbl)
            n96 = Wait (ms)(milliseconds to wait=u32 50) -> ()  [unwired: 1 out]
            n97 = Less?(x=w282, y=3.0) -> (x < y?=w280:bool)
            n98 = call-poly <vilib>:"NT Write Value.vi"("Numeric Array"=w287, "Name"=w286) -> ()  [unwired: 9 in, 1 out]
          }
        }
        frame #2 {
          # "stand still"
          n99 = call-poly <vilib>:"WPI_RobotDriveArcadeDrive.vi"("Y axis value"=0.0 ("X axis value"), "X axis value"=0.0, "RobotDriveDevRef"=w299) -> ("Motor Values"=w303:dbl[], "RobotDriveDevRef"=w298:T5)  [unwired: 1 in, 6 out]
          n100 = call-poly <vilib>:"NT Write Value.vi"("Numeric Array"=w303, "Name"=w300) -> ()  [unwired: 9 in, 1 out]
        }
        frame #3 {
          n101 = Tick Count (ms)() -> (millisecond timer value=w314:u32)
          n102 = while {
            tunnel: w315 -> [w342]
            tunnel: w314 -> [w340]
            tunnel: w313 -> [w329]
            tunnel: w312 -> [w334]
            tunnel: [w333] -> w311
            tunnel: [w329] -> w310
            tunnel: 7.0 ("setpoint") -> [w324]
            tunnel: w308 -> [w323]
            stop <- w326 continue-if-true
            w332 = u32 50 ("milliseconds to wait")
            # "Drive straight until close to wall, 4s timeout"
            n103 = call <vilib>:"ADI_IMU_ADIS16448_Get Angles.vi"("ADI IMU Interrupt DevRef"=w323) -> ("IMU Angles Out"=w318:T23)  [unwired: 7 in, 3 out]
            n104 = call-poly <vilib>:"WPI_UltrasonicGetRange.vi"("SonarMB1010AnalogDevRef"=w342) -> ("Distance"=w336:dbl)  [unwired: 8 in, 2 out]
            n105 = Wait (ms)(milliseconds to wait=w332) -> ()  [unwired: 1 out]
            n106 = Unbundle By Name(w318) -> ("Z Angle"=w317:dbl)
            n107 = Divide(x=w332, y=u32 1000) -> (x/y=w330:dbl)
            n108 = call-poly <vilib>:"PID.vi"("output range"=cluster{"output high":dbl, "output low":dbl} {"output high"=-0.7, "output low"=0.0}, "dt (s)"=w330, "PID gains"=T22 {"proportional gain (Kc)"=0.03, "integral time (Ti, min)"=0.0, "derivative time (Td, min)"=0.0003}, "process variable"=w336, "setpoint"=w324) -> ("output"=w316:dbl)  [unwired: 5 in, 1 out]
            n109 = Add(x=w340, y=u32 4000) -> (x+y=w328:u32)
            n110 = call-poly <vilib>:"PID.vi"("output range"=cluster{"output high":dbl, "output low":dbl} {"output high"=0.5, "output low"=-0.5}, "PID gains"=T22 {"proportional gain (Kc)"=0.1, "integral time (Ti, min)"=0.0, "derivative time (Td, min)"=0.0}, "process variable"=w317, "setpoint"=0.0) -> ("output"=w320:dbl)  [unwired: 6 in, 1 out]
            n111 = Tick Count (ms)() -> (millisecond timer value=w327:u32)
            n112 = Greater?(x=w328, y=w327) -> (0:w325:bool)
            n113 = call-poly <vilib>:"WPI_RobotDriveArcadeDrive.vi"("Y axis value"=w316, "X axis value"=w320, "RobotDriveDevRef"=w334) -> ("Motor Values"=w335:dbl[], "RobotDriveDevRef"=w333:T5)  [unwired: 6 in, 1 out]
            n114 = Greater?(x=w336, y=w324) -> (0:w341:bool)
            n115 = And(x=w325, y=w341) -> (x .and. y?=w326:bool)
            n116 = call-poly <vilib>:"NT Write Value.vi"("Numeric Array"=w335, "Name"=w329) -> ()  [unwired: 9 in, 1 out]
          }
        }
        frame #4 {
          # "Stop"
          n117 = call-poly <vilib>:"WPI_RobotDriveArcadeDrive.vi"("Y axis value"=0.0, "X axis value"=0.0, "RobotDriveDevRef"=w351) -> ("Motor Values"=w350:dbl[], "RobotDriveDevRef"=w345:T5)  [unwired: 6 in, 1 out]
          n118 = call-poly <vilib>:"NT Write Value.vi"("Numeric Array"=w350, "Name"=w347) -> ()  [unwired: 9 in, 1 out]
          n119 = call <vilib>:"WPI_RobotDriveDelayAndUpdateSafety.vi"("Delay (s)"=1.0, "RobotDriveDevRef"=w345) -> ("RobotDriveDevRef 2"=w344:T5)  [unwired: 8 in, 1 out]
        }
        frame #5 {
          n120 = call-poly <vilib>:"WPI_SolenoidSet.vi"("Value"=WPI_SolenoidValue."Forward", "SolenoidDevRef"=w355) -> ("SolenoidDevRef"=w354:T13)  [unwired: 8 in, 1 out]
          n121 = Wait (ms)(milliseconds to wait=u32 1000) -> ()  [unwired: 1 out]
        }
        frame #6 {
          n122 = call-poly <vilib>:"WPI_RobotDriveArcadeDrive.vi"("Y axis value"=0.7 ("X axis value"), "X axis value"=0.0, "RobotDriveDevRef"=w360) -> ("Motor Values"=w365:dbl[], "RobotDriveDevRef"=w362:T5)  [unwired: 1 in, 6 out]
          n123 = call <vilib>:"WPI_RobotDriveDelayAndUpdateSafety.vi"("Delay (s)"=1.0, "RobotDriveDevRef"=w362) -> ("RobotDriveDevRef 2"=w359:T5)  [unwired: 8 in, 1 out]
          n124 = call-poly <vilib>:"NT Write Value.vi"("Numeric Array"=w365, "Name"=w358) -> ()  [unwired: 9 in, 1 out]
        }
        frame #7 {
          n125 = call-poly <vilib>:"WPI_RobotDriveArcadeDrive.vi"("Y axis value"=0.0 ("X axis value"), "X axis value"=0.0, "RobotDriveDevRef"=w369) -> ("Motor Values"=w374:dbl[], "RobotDriveDevRef"=w372:T5)  [unwired: 1 in, 6 out]
          n126 = call-poly <vilib>:"NT Write Value.vi"("Numeric Array"=w374, "Name"=w367) -> ()  [unwired: 9 in, 1 out]
          n127 = call <vilib>:"WPI_RobotDriveDelayAndUpdateSafety.vi"("Delay (s)"=1.0, "RobotDriveDevRef"=w372) -> ("RobotDriveDevRef 2"=w368:T5)  [unwired: 8 in, 1 out]
        }
        frame #8 {
          n128 = call-poly <vilib>:"WPI_SolenoidSet.vi"("Value"=WPI_SolenoidValue."Reverse", "SolenoidDevRef"=w376) -> ()  [unwired: 8 in, 2 out]
        }
      }
      n129 = call <vilib>:"WPI_RobotDriveSafetyConfig.vi"("mode"=WPI_SafetyOutputConfigMenu."Enable", "RobotDriveDevRef"=w248) -> ()  [unwired: 8 in, 2 out]
    }
    frame "Left Gear no drop gear" {
      n130 = call <vilib>:"ADI_IMU_ADIS16448_Reset.vi"("ADI IMU Interrupt DevRef"=w407) -> ("ADI IMU Interrupt DevRef Out"=w405:T15)  [unwired: 9 in, 1 out]
      n131 = call <vilib>:"WPI_RobotDriveSafetyConfig.vi"("mode"=WPI_SafetyOutputConfigMenu."Disable", "RobotDriveDevRef"=w402) -> ("RobotDriveDevRef"=w401:T5)  [unwired: 8 in, 1 out]
      n132 = flat-sequence {
        tunnel: w403 -> [w422]
        tunnel: w401 -> [w412]
        tunnel: w404 -> [w411]
        tunnel: w405 -> [w423]
        tunnel: w406 -> [w424]
        tunnel: [w424] -> w385
        tunnel: [w423] -> w384
        tunnel: [w411] -> w383
        tunnel: [w409] -> w382
        tunnel: [w422] -> w381
        tunnel: [w432] -> w390
        tunnel: [w427] -> w389
        tunnel: [w425] -> w388
        tunnel: [w429] -> w387
        tunnel: [w431] -> w386
        tunnel: w385 -> [w432]
        tunnel: w384 -> [w428]
        tunnel: w383 -> [w426]
        tunnel: w382 -> [w430]
        tunnel: w381 -> [w431]
        tunnel: [w459] -> w395
        tunnel: [w458] -> w394
        tunnel: [w453] -> w393
        tunnel: [w451] -> w392
        tunnel: [w457] -> w391
        tunnel: w390 -> [w459]
        tunnel: w389 -> [w458]
        tunnel: w388 -> [w453]
        tunnel: w387 -> [w452]
        tunnel: w386 -> [w457]
        tunnel: [w464] -> w398
        tunnel: [w463] -> w397
        tunnel: [w460] -> w396
        tunnel: w395 -> [w468]
        tunnel: w394 -> [w461]
        tunnel: w393 -> [w466]
        tunnel: w392 -> [w465]
        tunnel: w391 -> [w460]
        tunnel: [w504] -> w380
        tunnel: w396 -> [w497]
        tunnel: w397 -> [w496]
        tunnel: w398 -> [w503]
        tunnel: [w497] -> _
        tunnel: [w496] -> _
        frame #0 {
          # "stand still"
          # "Drive straight (timed)\n\n** The idea here is to get the robot to the Baseline and stop. Tune as necessary"
          n133 = call-poly <vilib>:"WPI_RobotDriveArcadeDrive.vi"("Y axis value"=-0.7 ("X axis value"), "X axis value"=0.0, "RobotDriveDevRef"=w412) -> ("Motor Values"=w421:dbl[], "RobotDriveDevRef"=w415:T5)  [unwired: 1 in, 6 out]
          n134 = call-poly <vilib>:"NT Write Value.vi"("Numeric Array"=w421, "Name"=w411) -> ()  [unwired: 9 in, 1 out]
          n135 = call <vilib>:"WPI_RobotDriveDelayAndUpdateSafety.vi"("Delay (s)"=2.0, "RobotDriveDevRef"=w415) -> ("RobotDriveDevRef 2"=w413:T5)  [unwired: 8 in, 1 out]
          n136 = call-poly <vilib>:"WPI_RobotDriveArcadeDrive.vi"("Y axis value"=0.0 ("X axis value"), "X axis value"=0.0, "RobotDriveDevRef"=w413) -> ("Motor Values"=w420:dbl[], "RobotDriveDevRef"=w410:T5)  [unwired: 1 in, 6 out]
          n137 = call-poly <vilib>:"NT Write Value.vi"("Numeric Array"=w420, "Name"=w411) -> ()  [unwired: 9 in, 1 out]
          n138 = call <vilib>:"WPI_RobotDriveDelayAndUpdateSafety.vi"("Delay (s)"=1.0, "RobotDriveDevRef"=w410) -> ("RobotDriveDevRef 2"=w409:T5)  [unwired: 8 in, 1 out]
        }
        frame #1 {
          # "Turn left 45 deg, +/- 3 deg, no timeout"
          n139 = while {
            shift-right: [w448] -> w429
            shift-left: w430 -> [w449]
            shift-right: [w445] -> w427
            shift-left: w428 -> [w446]
            tunnel: w426 -> [w439]
            tunnel: [w439] -> w425
            stop <- w433 stop-if-true
            w437 = -45.0 ("setpoint")
            n140 = call <vilib>:"ADI_IMU_ADIS16448_Get Angles.vi"("ADI IMU Interrupt DevRef"=w446) -> ("IMU Angles Out"=w447:T23, "ADI IMU Interrupt DevRef Out"=w445:T15)  [unwired: 7 in, 2 out]
            n141 = Unbundle By Name(w447) -> ("Z Angle"=w438:dbl)
            n142 = call-poly <vilib>:"PID.vi"("output range"=cluster{"output high":dbl, "output low":dbl} {"output high"=0.6, "output low"=-0.6}, "PID gains"=T22 {"proportional gain (Kc)"=1.0, "integral time (Ti, min)"=0.0, "derivative time (Td, min)"=0.0}, "process variable"=w438, "setpoint"=w437) -> ("output"=w442:dbl)  [unwired: 6 in, 1 out]
            n143 = Subtract(x=w438, y=w437) -> (x-y=w436:dbl)
            n144 = call-poly <vilib>:"WPI_RobotDriveArcadeDrive.vi"("Y axis value"=0.0, "X axis value"=w442, "RobotDriveDevRef"=w449) -> ("Motor Values"=w440:dbl[], "RobotDriveDevRef"=w448:T5)  [unwired: 6 in, 1 out]
            n145 = Absolute Value(x=w436) -> (abs(x)=w435:dbl)
            n146 = Wait (ms)(milliseconds to wait=u32 50) -> ()  [unwired: 1 out]
            n147 = Less?(x=w435, y=3.0) -> (x < y?=w433:bool)
            n148 = call-poly <vilib>:"NT Write Value.vi"("Numeric Array"=w440, "Name"=w439) -> ()  [unwired: 9 in, 1 out]
          }
        }
        frame #2 {
          # "stand still"
          n149 = call-poly <vilib>:"WPI_RobotDriveArcadeDrive.vi"("Y axis value"=0.0 ("X axis value"), "X axis value"=0.0, "RobotDriveDevRef"=w452) -> ("Motor Values"=w456:dbl[], "RobotDriveDevRef"=w451:T5)  [unwired: 1 in, 6 out]
          n150 = call-poly <vilib>:"NT Write Value.vi"("Numeric Array"=w456, "Name"=w453) -> ()  [unwired: 9 in, 1 out]
        }
        frame #3 {
          n151 = Tick Count (ms)() -> (millisecond timer value=w467:u32)
          n152 = while {
            tunnel: w468 -> [w495]
            tunnel: w467 -> [w493]
            tunnel: w466 -> [w482]
            tunnel: w465 -> [w487]
            tunnel: [w486] -> w464
            tunnel: [w482] -> w463
            tunnel: 7.0 ("setpoint") -> [w477]
            tunnel: w461 -> [w476]
            stop <- w479 continue-if-true
            w485 = u32 50 ("milliseconds to wait")
            # "Drive straight until close to wall, 3s timeout"
            n153 = call <vilib>:"ADI_IMU_ADIS16448_Get Angles.vi"("ADI IMU Interrupt DevRef"=w476) -> ("IMU Angles Out"=w471:T23)  [unwired: 7 in, 3 out]
            n154 = call-poly <vilib>:"WPI_UltrasonicGetRange.vi"("SonarMB1010AnalogDevRef"=w495) -> ("Distance"=w489:dbl)  [unwired: 8 in, 2 out]
            n155 = Wait (ms)(milliseconds to wait=w485) -> ()  [unwired: 1 out]
            n156 = Unbundle By Name(w471) -> ("Z Angle"=w470:dbl)
            n157 = Divide(x=w485, y=u32 1000) -> (x/y=w483:dbl)
            n158 = call-poly <vilib>:"PID.vi"("output range"=cluster{"output high":dbl, "output low":dbl} {"output high"=-0.7, "output low"=0.0}, "dt (s)"=w483, "PID gains"=T22 {"proportional gain (Kc)"=0.03, "integral time (Ti, min)"=0.0, "derivative time (Td, min)"=0.0003}, "process variable"=w489, "setpoint"=w477) -> ("output"=w469:dbl)  [unwired: 5 in, 1 out]
            n159 = Add(x=w493, y=u32 3000) -> (x+y=w481:u32)
            n160 = call-poly <vilib>:"PID.vi"("output range"=cluster{"output high":dbl, "output low":dbl} {"output high"=0.5, "output low"=-0.5}, "PID gains"=T22 {"proportional gain (Kc)"=0.1, "integral time (Ti, min)"=0.0, "derivative time (Td, min)"=0.0}, "process variable"=w470, "setpoint"=0.0) -> ("output"=w473:dbl)  [unwired: 6 in, 1 out]
            n161 = Tick Count (ms)() -> (millisecond timer value=w480:u32)
            n162 = Greater?(x=w481, y=w480) -> (0:w478:bool)
            n163 = call-poly <vilib>:"WPI_RobotDriveArcadeDrive.vi"("Y axis value"=w469, "X axis value"=w473, "RobotDriveDevRef"=w487) -> ("Motor Values"=w488:dbl[], "RobotDriveDevRef"=w486:T5)  [unwired: 6 in, 1 out]
            n164 = Greater?(x=w489, y=w477) -> (0:w494:bool)
            n165 = And(x=w478, y=w494) -> (x .and. y?=w479:bool)
            n166 = call-poly <vilib>:"NT Write Value.vi"("Numeric Array"=w488, "Name"=w482) -> ()  [unwired: 9 in, 1 out]
          }
        }
        frame #4 {
          # "Stop"
          n167 = call-poly <vilib>:"WPI_RobotDriveArcadeDrive.vi"("Y axis value"=0.0, "X axis value"=0.0, "RobotDriveDevRef"=w503) -> ("Motor Values"=w502:dbl[], "RobotDriveDevRef"=w499:T5)  [unwired: 6 in, 1 out]
          n168 = call-poly <vilib>:"NT Write Value.vi"("Numeric Array"=w502, "Name"=w496) -> ()  [unwired: 9 in, 1 out]
          n169 = call <vilib>:"WPI_RobotDriveDelayAndUpdateSafety.vi"("Delay (s)"=1.0, "RobotDriveDevRef"=w499) -> ("RobotDriveDevRef 2"=w504:T5)  [unwired: 8 in, 1 out]
        }
      }
      n170 = call <vilib>:"WPI_RobotDriveSafetyConfig.vi"("mode"=WPI_SafetyOutputConfigMenu."Enable", "RobotDriveDevRef"=w380) -> ()  [unwired: 8 in, 2 out]
    }
    frame "Right Gear" {
      n171 = call <vilib>:"ADI_IMU_ADIS16448_Reset.vi"("ADI IMU Interrupt DevRef"=w557) -> ("ADI IMU Interrupt DevRef Out"=w555:T15)  [unwired: 9 in, 1 out]
      n172 = call <vilib>:"WPI_RobotDriveSafetyConfig.vi"("mode"=WPI_SafetyOutputConfigMenu."Disable", "RobotDriveDevRef"=w552) -> ("RobotDriveDevRef"=w551:T5)  [unwired: 8 in, 1 out]
      n173 = flat-sequence {
        tunnel: w553 -> [w571]
        tunnel: w551 -> [w561]
        tunnel: w554 -> [w560]
        tunnel: w555 -> [w572]
        tunnel: w556 -> [w573]
        tunnel: [w573] -> w525
        tunnel: [w572] -> w524
        tunnel: [w560] -> w523
        tunnel: [w559] -> w522
        tunnel: [w571] -> w521
        tunnel: w520 -> [w558]
        tunnel: [w558] -> w519
        tunnel: [w582] -> w530
        tunnel: [w577] -> w529
        tunnel: [w575] -> w528
        tunnel: [w579] -> w527
        tunnel: [w581] -> w526
        tunnel: w525 -> [w582]
        tunnel: w524 -> [w578]
        tunnel: w523 -> [w576]
        tunnel: w522 -> [w580]
        tunnel: w521 -> [w581]
        tunnel: w519 -> [w574]
        tunnel: [w574] -> w518
        tunnel: [w610] -> w535
        tunnel: [w609] -> w534
        tunnel: [w604] -> w533
        tunnel: [w602] -> w532
        tunnel: [w608] -> w531
        tunnel: w530 -> [w610]
        tunnel: w529 -> [w609]
        tunnel: w528 -> [w604]
        tunnel: w527 -> [w603]
        tunnel: w526 -> [w608]
        tunnel: w518 -> [w601]
        tunnel: [w601] -> w517
        tunnel: [w616] -> w547
        tunnel: [w615] -> w546
        tunnel: [w612] -> w543
        tunnel: w535 -> [w620]
        tunnel: w534 -> [w613]
        tunnel: w533 -> [w618]
        tunnel: w532 -> [w617]
        tunnel: w531 -> [w612]
        tunnel: w517 -> [w611]
        tunnel: [w611] -> w516
        tunnel: w547 -> [w657]
        tunnel: w546 -> [w653]
        tunnel: [w650] -> w545
        tunnel: [w653] -> w544
        tunnel: w543 -> [w652]
        tunnel: [w652] -> w542
        tunnel: w516 -> [w648]
        tunnel: [w648] -> w515
        tunnel: w545 -> [w664]
        tunnel: w544 -> [w663]
        tunnel: w542 -> [w662]
        tunnel: [w664] -> w514
        tunnel: [w663] -> w512
        tunnel: [w661] -> w510
        tunnel: w515 -> [w658]
        tunnel: [w658] -> w508
        tunnel: w514 -> [w671]
        tunnel: [w671] -> w513
        tunnel: w512 -> [w670]
        tunnel: [w670] -> w511
        tunnel: w510 -> [w669]
        tunnel: [w669] -> w509
        tunnel: w508 -> [w668]
        tunnel: [w667] -> w507
        tunnel: w513 -> [w677]
        tunnel: w511 -> [w675]
        tunnel: w509 -> [w683]
        tunnel: [w676] -> w541
        tunnel: [w675] -> w540
        tunnel: [w683] -> w539
        tunnel: w507 -> [w674]
        tunnel: [w672] -> w506
        tunnel: w541 -> [w687]
        tunnel: w540 -> [w685]
        tunnel: w539 -> [w693]
        tunnel: [w686] -> w538
        tunnel: [w685] -> w537
        tunnel: [w693] -> w536
        tunnel: w506 -> [w684]
        tunnel: [w684] -> w505
        tunnel: [w697] -> _
        tunnel: [w698] -> w549
        tunnel: w538 -> [w698]
        tunnel: w537 -> [w697]
        tunnel: w536 -> [w695]
        tunnel: [w694] -> _
        tunnel: w505 -> [w694]
        frame #0 {
          # "stand still"
          # "Drive straight (timed)"
          n174 = call-poly <vilib>:"WPI_RobotDriveArcadeDrive.vi"("Y axis value"=-0.85 ("X axis value"), "X axis value"=0.0, "RobotDriveDevRef"=w561) -> ("Motor Values"=w570:dbl[], "RobotDriveDevRef"=w564:T5)  [unwired: 1 in, 6 out]
          n175 = call-poly <vilib>:"NT Write Value.vi"("Numeric Array"=w570, "Name"=w560) -> ()  [unwired: 9 in, 1 out]
          n176 = call <vilib>:"WPI_RobotDriveDelayAndUpdateSafety.vi"("Delay (s)"=2.0, "RobotDriveDevRef"=w564) -> ("RobotDriveDevRef 2"=w562:T5)  [unwired: 8 in, 1 out]
          n177 = call-poly <vilib>:"WPI_RobotDriveArcadeDrive.vi"("Y axis value"=0.0 ("X axis value"), "X axis value"=0.0, "RobotDriveDevRef"=w562) -> ("Motor Values"=w569:dbl[], "RobotDriveDevRef"=w559:T5)  [unwired: 1 in, 6 out]
          n178 = call-poly <vilib>:"NT Write Value.vi"("Numeric Array"=w569, "Name"=w560) -> ()  [unwired: 9 in, 1 out]
        }
        frame #1 {
          # "Turn left 45 deg"
          n179 = while {
            shift-right: [w598] -> w579
            shift-left: w580 -> [w599]
            shift-right: [w595] -> w577
            shift-left: w578 -> [w596]
            tunnel: w576 -> [w589]
            tunnel: [w589] -> w575
            stop <- w583 stop-if-true
            w587 = 45.0 ("setpoint")
            n180 = call <vilib>:"ADI_IMU_ADIS16448_Get Angles.vi"("ADI IMU Interrupt DevRef"=w596) -> ("IMU Angles Out"=w597:T23, "ADI IMU Interrupt DevRef Out"=w595:T15)  [unwired: 7 in, 2 out]
            n181 = Unbundle By Name(w597) -> ("Z Angle"=w588:dbl)
            n182 = call-poly <vilib>:"PID.vi"("output range"=cluster{"output high":dbl, "output low":dbl} {"output high"=0.6, "output low"=-0.6}, "PID gains"=T22 {"proportional gain (Kc)"=0.1, "integral time (Ti, min)"=0.0, "derivative time (Td, min)"=0.0}, "process variable"=w588, "setpoint"=w587) -> ("output"=w592:dbl)  [unwired: 6 in, 1 out]
            n183 = Subtract(x=w588, y=w587) -> (x-y=w586:dbl)
            n184 = call-poly <vilib>:"WPI_RobotDriveArcadeDrive.vi"("Y axis value"=0.0, "X axis value"=w592, "RobotDriveDevRef"=w599) -> ("Motor Values"=w590:dbl[], "RobotDriveDevRef"=w598:T5)  [unwired: 6 in, 1 out]
            n185 = Absolute Value(x=w586) -> (abs(x)=w585:dbl)
            n186 = Wait (ms)(milliseconds to wait=u32 50) -> ()  [unwired: 1 out]
            n187 = Less?(x=w585, y=3.0) -> (x < y?=w583:bool)
            n188 = call-poly <vilib>:"NT Write Value.vi"("Numeric Array"=w590, "Name"=w589) -> ()  [unwired: 9 in, 1 out]
          }
        }
        frame #2 {
          # "stand still"
          n189 = call-poly <vilib>:"WPI_RobotDriveArcadeDrive.vi"("Y axis value"=0.0 ("X axis value"), "X axis value"=0.0, "RobotDriveDevRef"=w603) -> ("Motor Values"=w607:dbl[], "RobotDriveDevRef"=w602:T5)  [unwired: 1 in, 6 out]
          n190 = call-poly <vilib>:"NT Write Value.vi"("Numeric Array"=w607, "Name"=w604) -> ()  [unwired: 9 in, 1 out]
        }
        frame #3 {
          n191 = Tick Count (ms)() -> (millisecond timer value=w619:u32)
          n192 = while {
            tunnel: w620 -> [w647]
            tunnel: w619 -> [w645]
            tunnel: w618 -> [w634]
            tunnel: w617 -> [w639]
            tunnel: [w638] -> w616
            tunnel: [w634] -> w615
            tunnel: 7.0 ("setpoint") -> [w629]
            tunnel: w613 -> [w628]
            stop <- w631 continue-if-true
            w637 = u32 50 ("milliseconds to wait")
            # "Drive straight until close to wall, 4s timeout"
            n193 = call <vilib>:"ADI_IMU_ADIS16448_Get Angles.vi"("ADI IMU Interrupt DevRef"=w628) -> ("IMU Angles Out"=w623:T23)  [unwired: 7 in, 3 out]
            n194 = call-poly <vilib>:"WPI_UltrasonicGetRange.vi"("SonarMB1010AnalogDevRef"=w647) -> ("Distance"=w641:dbl)  [unwired: 8 in, 2 out]
            n195 = Wait (ms)(milliseconds to wait=w637) -> ()  [unwired: 1 out]
            n196 = Unbundle By Name(w623) -> ("Z Angle"=w622:dbl)
            n197 = Divide(x=w637, y=u32 1000) -> (x/y=w635:dbl)
            n198 = call-poly <vilib>:"PID.vi"("output range"=cluster{"output high":dbl, "output low":dbl} {"output high"=-0.7, "output low"=0.0}, "dt (s)"=w635, "PID gains"=T22 {"proportional gain (Kc)"=0.03, "integral time (Ti, min)"=0.0, "derivative time (Td, min)"=0.0003}, "process variable"=w641, "setpoint"=w629) -> ("output"=w621:dbl)  [unwired: 5 in, 1 out]
            n199 = Add(x=w645, y=u32 4000) -> (x+y=w633:u32)
            n200 = call-poly <vilib>:"PID.vi"("output range"=cluster{"output high":dbl, "output low":dbl} {"output high"=0.5, "output low"=-0.5}, "PID gains"=T22 {"proportional gain (Kc)"=0.1, "integral time (Ti, min)"=0.0, "derivative time (Td, min)"=0.0}, "process variable"=w622, "setpoint"=0.0) -> ("output"=w625:dbl)  [unwired: 6 in, 1 out]
            n201 = Tick Count (ms)() -> (millisecond timer value=w632:u32)
            n202 = Greater?(x=w633, y=w632) -> (0:w630:bool)
            n203 = call-poly <vilib>:"WPI_RobotDriveArcadeDrive.vi"("Y axis value"=w621, "X axis value"=w625, "RobotDriveDevRef"=w639) -> ("Motor Values"=w640:dbl[], "RobotDriveDevRef"=w638:T5)  [unwired: 6 in, 1 out]
            n204 = Greater?(x=w641, y=w629) -> (0:w646:bool)
            n205 = And(x=w630, y=w646) -> (x .and. y?=w631:bool)
            n206 = call-poly <vilib>:"NT Write Value.vi"("Numeric Array"=w640, "Name"=w634) -> ()  [unwired: 9 in, 1 out]
          }
        }
        frame #4 {
          # "Stop"
          n207 = call-poly <vilib>:"WPI_RobotDriveArcadeDrive.vi"("Y axis value"=0.0, "X axis value"=0.0, "RobotDriveDevRef"=w657) -> ("Motor Values"=w656:dbl[], "RobotDriveDevRef"=w651:T5)  [unwired: 6 in, 1 out]
          n208 = call-poly <vilib>:"NT Write Value.vi"("Numeric Array"=w656, "Name"=w653) -> ()  [unwired: 9 in, 1 out]
          n209 = call <vilib>:"WPI_RobotDriveDelayAndUpdateSafety.vi"("Delay (s)"=1.0, "RobotDriveDevRef"=w651) -> ("RobotDriveDevRef 2"=w650:T5)  [unwired: 8 in, 1 out]
        }
        frame #5 {
          # "Open Gear"
          n210 = call-poly <vilib>:"WPI_SolenoidSet.vi"("Value"=WPI_SolenoidValue."Forward", "SolenoidDevRef"=w662) -> ("SolenoidDevRef"=w661:T13)  [unwired: 8 in, 1 out]
          n211 = Wait (ms)(milliseconds to wait=u32 500) -> ()  [unwired: 1 out]
        }
        frame #6 {
          # "Push"
          n212 = Wait (ms)(milliseconds to wait=u32 2000) -> ()  [unwired: 1 out]
          n213 = call-poly <vilib>:"WPI_SolenoidSet.vi"("Value"=WPI_SolenoidValue."Forward", "SolenoidDevRef"=w668) -> ("SolenoidDevRef"=w667:T13)  [unwired: 8 in, 1 out]
        }
        frame #7 {
          # "Retract pusher"
          n214 = call-poly <vilib>:"WPI_RobotDriveArcadeDrive.vi"("Y axis value"=0.7 ("X axis value"), "X axis value"=0.0, "RobotDriveDevRef"=w677) -> ("Motor Values"=w682:dbl[], "RobotDriveDevRef"=w679:T5)  [unwired: 1 in, 6 out]
          n215 = call-poly <vilib>:"WPI_SolenoidSet.vi"("Value"=WPI_SolenoidValue."Reverse", "SolenoidDevRef"=w674) -> ("SolenoidDevRef"=w672:T13)  [unwired: 8 in, 1 out]
          n216 = call <vilib>:"WPI_RobotDriveDelayAndUpdateSafety.vi"("Delay (s)"=1.0, "RobotDriveDevRef"=w679) -> ("RobotDriveDevRef 2"=w676:T5)  [unwired: 8 in, 1 out]
          n217 = call-poly <vilib>:"NT Write Value.vi"("Numeric Array"=w682, "Name"=w675) -> ()  [unwired: 9 in, 1 out]
        }
        frame #8 {
          n218 = call-poly <vilib>:"WPI_RobotDriveArcadeDrive.vi"("Y axis value"=0.0 ("X axis value"), "X axis value"=0.0, "RobotDriveDevRef"=w687) -> ("Motor Values"=w692:dbl[], "RobotDriveDevRef"=w690:T5)  [unwired: 1 in, 6 out]
          n219 = call-poly <vilib>:"NT Write Value.vi"("Numeric Array"=w692, "Name"=w685) -> ()  [unwired: 9 in, 1 out]
          n220 = call <vilib>:"WPI_RobotDriveDelayAndUpdateSafety.vi"("Delay (s)"=1.0, "RobotDriveDevRef"=w690) -> ("RobotDriveDevRef 2"=w686:T5)  [unwired: 8 in, 1 out]
        }
        frame #9 {
          n221 = call-poly <vilib>:"WPI_SolenoidSet.vi"("Value"=WPI_SolenoidValue."Reverse", "SolenoidDevRef"=w695) -> ()  [unwired: 8 in, 2 out]
        }
      }
      n222 = call <vilib>:"WPI_RobotDriveSafetyConfig.vi"("mode"=WPI_SafetyOutputConfigMenu."Enable", "RobotDriveDevRef"=w549) -> ()  [unwired: 8 in, 2 out]
    }
    frame "Right Gear no drop gear" {
      n223 = call <vilib>:"ADI_IMU_ADIS16448_Reset.vi"("ADI IMU Interrupt DevRef"=w726) -> ("ADI IMU Interrupt DevRef Out"=w724:T15)  [unwired: 9 in, 1 out]
      n224 = call <vilib>:"WPI_RobotDriveSafetyConfig.vi"("mode"=WPI_SafetyOutputConfigMenu."Disable", "RobotDriveDevRef"=w721) -> ("RobotDriveDevRef"=w720:T5)  [unwired: 8 in, 1 out]
      n225 = flat-sequence {
        tunnel: w722 -> [w741]
        tunnel: w720 -> [w731]
        tunnel: w723 -> [w730]
        tunnel: w724 -> [w742]
        tunnel: w725 -> [w743]
        tunnel: [w743] -> w704
        tunnel: [w742] -> w703
        tunnel: [w730] -> w702
        tunnel: [w728] -> w701
        tunnel: [w741] -> w700
        tunnel: [w751] -> w709
        tunnel: [w746] -> w708
        tunnel: [w744] -> w707
        tunnel: [w748] -> w706
        tunnel: [w750] -> w705
        tunnel: w704 -> [w751]
        tunnel: w703 -> [w747]
        tunnel: w702 -> [w745]
        tunnel: w701 -> [w749]
        tunnel: w700 -> [w750]
        tunnel: [w778] -> w714
        tunnel: [w777] -> w713
        tunnel: [w772] -> w712
        tunnel: [w770] -> w711
        tunnel: [w776] -> w710
        tunnel: w709 -> [w778]
        tunnel: w708 -> [w777]
        tunnel: w707 -> [w772]
        tunnel: w706 -> [w771]
        tunnel: w705 -> [w776]
        tunnel: [w783] -> w717
        tunnel: [w782] -> w716
        tunnel: [w779] -> w715
        tunnel: w714 -> [w787]
        tunnel: w713 -> [w780]
        tunnel: w712 -> [w785]
        tunnel: w711 -> [w784]
        tunnel: w710 -> [w779]
        tunnel: [w823] -> w699
        tunnel: w715 -> [w815]
        tunnel: w716 -> [w816]
        tunnel: w717 -> [w822]
        tunnel: [w816] -> _
        tunnel: [w815] -> _
        frame #0 {
          # "stand still"
          # "Drive straight (timed)"
          n226 = call-poly <vilib>:"WPI_RobotDriveArcadeDrive.vi"("Y axis value"=-0.7 ("X axis value"), "X axis value"=0.0, "RobotDriveDevRef"=w731) -> ("Motor Values"=w740:dbl[], "RobotDriveDevRef"=w734:T5)  [unwired: 1 in, 6 out]
          n227 = call-poly <vilib>:"NT Write Value.vi"("Numeric Array"=w740, "Name"=w730) -> ()  [unwired: 9 in, 1 out]
          n228 = call <vilib>:"WPI_RobotDriveDelayAndUpdateSafety.vi"("Delay (s)"=2.0, "RobotDriveDevRef"=w734) -> ("RobotDriveDevRef 2"=w732:T5)  [unwired: 8 in, 1 out]
          n229 = call-poly <vilib>:"WPI_RobotDriveArcadeDrive.vi"("Y axis value"=0.0 ("X axis value"), "X axis value"=0.0, "RobotDriveDevRef"=w732) -> ("Motor Values"=w739:dbl[], "RobotDriveDevRef"=w729:T5)  [unwired: 1 in, 6 out]
          n230 = call-poly <vilib>:"NT Write Value.vi"("Numeric Array"=w739, "Name"=w730) -> ()  [unwired: 9 in, 1 out]
          n231 = call <vilib>:"WPI_RobotDriveDelayAndUpdateSafety.vi"("Delay (s)"=1.0, "RobotDriveDevRef"=w729) -> ("RobotDriveDevRef 2"=w728:T5)  [unwired: 8 in, 1 out]
        }
        frame #1 {
          # "Turn left 45 deg"
          n232 = while {
            shift-right: [w767] -> w748
            shift-left: w749 -> [w768]
            shift-right: [w764] -> w746
            shift-left: w747 -> [w765]
            tunnel: w745 -> [w758]
            tunnel: [w758] -> w744
            stop <- w752 stop-if-true
            w756 = 45.0 ("setpoint")
            n233 = call <vilib>:"ADI_IMU_ADIS16448_Get Angles.vi"("ADI IMU Interrupt DevRef"=w765) -> ("IMU Angles Out"=w766:T23, "ADI IMU Interrupt DevRef Out"=w764:T15)  [unwired: 7 in, 2 out]
            n234 = Unbundle By Name(w766) -> ("Z Angle"=w757:dbl)
            n235 = call-poly <vilib>:"PID.vi"("output range"=cluster{"output high":dbl, "output low":dbl} {"output high"=0.6, "output low"=-0.6}, "PID gains"=T22 {"proportional gain (Kc)"=1.0, "integral time (Ti, min)"=0.0, "derivative time (Td, min)"=0.0}, "process variable"=w757, "setpoint"=w756) -> ("output"=w761:dbl)  [unwired: 6 in, 1 out]
            n236 = Subtract(x=w757, y=w756) -> (x-y=w755:dbl)
            n237 = call-poly <vilib>:"WPI_RobotDriveArcadeDrive.vi"("Y axis value"=0.0, "X axis value"=w761, "RobotDriveDevRef"=w768) -> ("Motor Values"=w759:dbl[], "RobotDriveDevRef"=w767:T5)  [unwired: 6 in, 1 out]
            n238 = Absolute Value(x=w755) -> (abs(x)=w754:dbl)
            n239 = Wait (ms)(milliseconds to wait=u32 50) -> ()  [unwired: 1 out]
            n240 = Less?(x=w754, y=2.0) -> (x < y?=w752:bool)
            n241 = call-poly <vilib>:"NT Write Value.vi"("Numeric Array"=w759, "Name"=w758) -> ()  [unwired: 9 in, 1 out]
          }
        }
        frame #2 {
          # "stand still"
          n242 = call-poly <vilib>:"WPI_RobotDriveArcadeDrive.vi"("Y axis value"=0.0 ("X axis value"), "X axis value"=0.0, "RobotDriveDevRef"=w771) -> ("Motor Values"=w775:dbl[], "RobotDriveDevRef"=w770:T5)  [unwired: 1 in, 6 out]
          n243 = call-poly <vilib>:"NT Write Value.vi"("Numeric Array"=w775, "Name"=w772) -> ()  [unwired: 9 in, 1 out]
        }
        frame #3 {
          n244 = Tick Count (ms)() -> (millisecond timer value=w786:u32)
          n245 = while {
            tunnel: w787 -> [w814]
            tunnel: w786 -> [w812]
            tunnel: w785 -> [w801]
            tunnel: w784 -> [w806]
            tunnel: [w805] -> w783
            tunnel: [w801] -> w782
            tunnel: 7.0 ("setpoint") -> [w796]
            tunnel: w780 -> [w795]
            stop <- w798 continue-if-true
            w804 = u32 50 ("milliseconds to wait")
            # "Drive straight until close to wall, 3s timeout"
            n246 = call <vilib>:"ADI_IMU_ADIS16448_Get Angles.vi"("ADI IMU Interrupt DevRef"=w795) -> ("IMU Angles Out"=w790:T23)  [unwired: 7 in, 3 out]
            n247 = call-poly <vilib>:"WPI_UltrasonicGetRange.vi"("SonarMB1010AnalogDevRef"=w814) -> ("Distance"=w808:dbl)  [unwired: 8 in, 2 out]
            n248 = Wait (ms)(milliseconds to wait=w804) -> ()  [unwired: 1 out]
            n249 = Unbundle By Name(w790) -> ("Z Angle"=w789:dbl)
            n250 = Divide(x=w804, y=u32 1000) -> (x/y=w802:dbl)
            n251 = call-poly <vilib>:"PID.vi"("output range"=cluster{"output high":dbl, "output low":dbl} {"output high"=-0.7, "output low"=0.0}, "dt (s)"=w802, "PID gains"=T22 {"proportional gain (Kc)"=0.03, "integral time (Ti, min)"=0.0, "derivative time (Td, min)"=0.0003}, "process variable"=w808, "setpoint"=w796) -> ("output"=w788:dbl)  [unwired: 5 in, 1 out]
            n252 = Add(x=w812, y=u32 3000) -> (x+y=w800:u32)
            n253 = call-poly <vilib>:"PID.vi"("output range"=cluster{"output high":dbl, "output low":dbl} {"output high"=0.5, "output low"=-0.5}, "PID gains"=T22 {"proportional gain (Kc)"=0.1, "integral time (Ti, min)"=0.0, "derivative time (Td, min)"=0.0}, "process variable"=w789, "setpoint"=45.0) -> ("output"=w792:dbl)  [unwired: 6 in, 1 out]
            n254 = Tick Count (ms)() -> (millisecond timer value=w799:u32)
            n255 = Greater?(x=w800, y=w799) -> (0:w797:bool)
            n256 = call-poly <vilib>:"WPI_RobotDriveArcadeDrive.vi"("Y axis value"=w788, "X axis value"=w792, "RobotDriveDevRef"=w806) -> ("Motor Values"=w807:dbl[], "RobotDriveDevRef"=w805:T5)  [unwired: 6 in, 1 out]
            n257 = Greater?(x=w808, y=w796) -> (0:w813:bool)
            n258 = And(x=w797, y=w813) -> (x .and. y?=w798:bool)
            n259 = call-poly <vilib>:"NT Write Value.vi"("Numeric Array"=w807, "Name"=w801) -> ()  [unwired: 9 in, 1 out]
          }
        }
        frame #4 {
          # "Stop"
          n260 = call-poly <vilib>:"WPI_RobotDriveArcadeDrive.vi"("Y axis value"=0.0, "X axis value"=0.0, "RobotDriveDevRef"=w822) -> ("Motor Values"=w821:dbl[], "RobotDriveDevRef"=w818:T5)  [unwired: 6 in, 1 out]
          n261 = call-poly <vilib>:"NT Write Value.vi"("Numeric Array"=w821, "Name"=w816) -> ()  [unwired: 9 in, 1 out]
          n262 = call <vilib>:"WPI_RobotDriveDelayAndUpdateSafety.vi"("Delay (s)"=1.0, "RobotDriveDevRef"=w818) -> ("RobotDriveDevRef 2"=w823:T5)  [unwired: 8 in, 1 out]
        }
      }
      n263 = call <vilib>:"WPI_RobotDriveSafetyConfig.vi"("mode"=WPI_SafetyOutputConfigMenu."Enable", "RobotDriveDevRef"=w699) -> ()  [unwired: 8 in, 2 out]
    }
  }
  n264 = while {
    stop <- FALSE stop-if-true
    n265 = call <vilib>:"WPI_DriverStationReport Robot Code State.vi"("Autonomous"=TRUE) -> ()  [unwired: 10 in, 1 out]
    n266 = Wait (ms)(milliseconds to wait=u32 20) -> ()  [unwired: 1 out]
  }
